vi "Read Self Queue.vi"(8 "error in (no error)":errorcluster, 11 "Generic Actor in":refnum<class "Generic Actor.lvclass">) -> (0 "error out":errorcluster, 2 "Self Enqueuer":refnum<class "Message Enqueuer.lvclass">, 3 "Generic Actor out":refnum<class "Generic Actor.lvclass">)   [LabVIEW 2020, in "Generic Actor.lvlib" / "Generic Actor.lvclass"]
uses:
  Generic Actor.lvclass
  C:/Program Files (x86)/National Instruments/LabVIEW 2020/vi.lib/ActorFramework/Actor/Actor.lvclass
  <vilib>/ActorFramework/Message Enqueuer/Message Enqueuer.lvclass
  <vilib>/ActorFramework/Actor/Actor.lvclass/Actor.ctl
  <vilib>/ActorFramework/Message Enqueuer/Message Enqueuer.lvclass/Message Enqueuer.ctl
  <vilib>/ActorFramework/Message Enqueuer/Init from Existing Queue.vi
  <vilib>/ActorFramework/Actor/Actor.lvclass
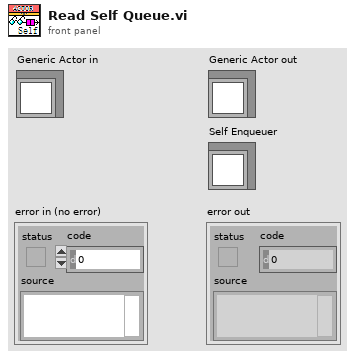
[diagram p1: front panel]
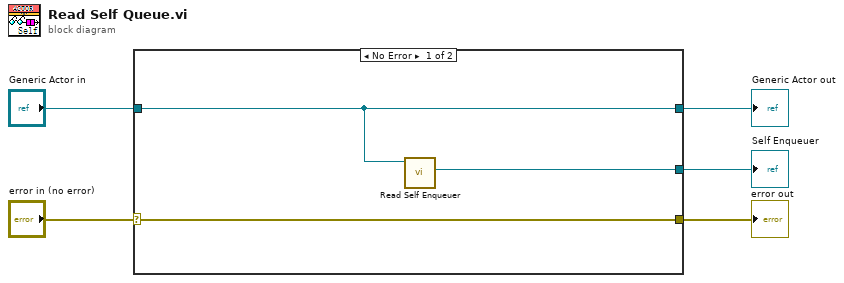
[diagram p0: block diagram]
diagram:
  n1 = case shown="No Error" "error in (no error)" {
    selector: "error in (no error)" -> [w8 w10]
    tunnel: [w8 w10] -> w4
    tunnel: [w7 w9] -> w2
    tunnel: "Generic Actor in" -> [w7 w9]
    tunnel: [w6 _] -> w1
    frame No Error {
      n2 = call <vilib>:"Read Self Enqueuer.vi"("Actor"=w7) -> ("Self Enqueuer"=w6:refnum<class "Message Enqueuer.lvclass">)  [unwired: 10 in]
    }
    frame Error {
    }
  }
  "error out" <- w4
  "Generic Actor out" <- w2
  "Self Enqueuer" <- w1
